vi "Pc Robo control.vi"() -> ()   [LabVIEW 2017]
uses:
  <vilib>/Utility/inputDevices.llb/joystickAcquire.vi
  <vilib>/Platform/NI_3dgraph.lvlib
panel:
  in  "error in (no error)":errorcluster
  in  "stop":bool
  out "error out":errorcluster
  out "Numeric":dbl
  out "Phi1":dbl
  out "K1":dbl
  out "Phi2":dbl
  out "K2":dbl
  out "L1":dbl(slide) scale=-0.09..0.09
  out "L2":dbl(slide) scale=-0.09..0.09
  out "L3":dbl(slide) scale=-0.09..0.09
  out "L4":dbl(slide) scale=-0.09..0.09
  out "L5":dbl(slide) scale=-0.09..0.09
  out "L6":dbl(slide) scale=-0.09..0.09
  in  "3D Curve":refnum<k7>(container)
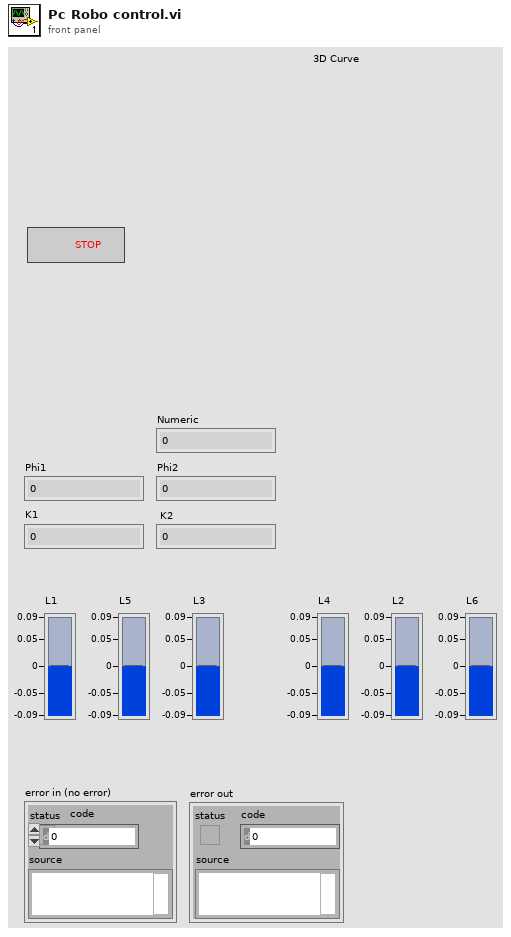
[diagram p1: front panel]
types:
  T1 = cluster{"X axis":i32, "Y axis":i32, "Z axis":i32, "X axis rotation":i32, "Y axis rotation":i32, "Z axis rotation":i32, "U axis":i32, "V axis":i32}
  T2 = cluster{"button 1":bool, "button 2":bool, "button 3":bool, "button 4":bool, "button 5":bool, "button 6":bool, "button 7":bool, "button 8":bool, "button 9":bool, "button 10":bool, "button 11":bool, "button 12":bool, "button 13":bool, "button 14":bool, "button 15":bool, "button 16":bool, "button 17":bool, "button 18":bool, "button 19":bool, "button 20":bool, "button 21":bool, "button 22":bool, "button 23":bool, "button 24":bool, "button 25":bool, "button 26":bool, "button 27":bool, "button 28":bool, "button 29":bool, "button 30":bool, "button 31":bool, "button 32":bool}
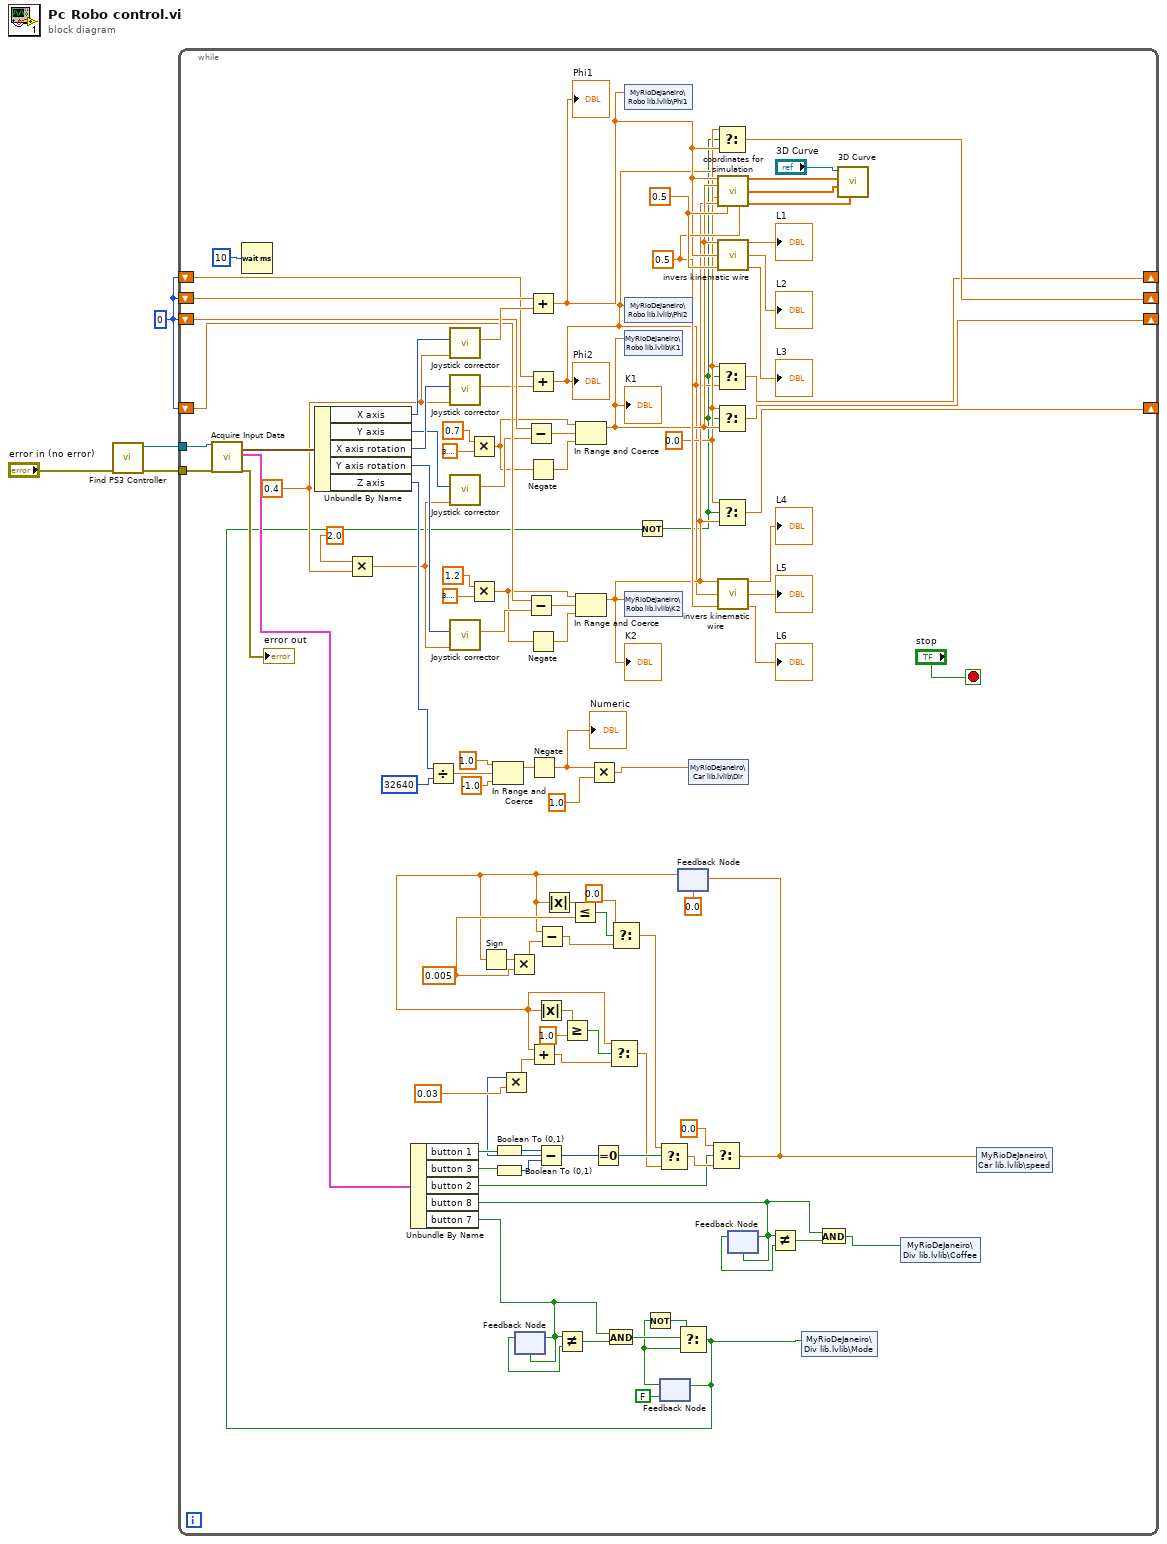
[diagram p0: block diagram]
diagram:
  w4 = 0
  n1 = call "Find PS3 Controller.vi"("error in (no error)"="error in (no error)") -> ("error out"=w2:errorcluster, "Controller Reference Out"=w3:refnum<k1>)  [unwired: 9 in]
  n2 = while {
    tunnel: w2 -> [w101]
    tunnel: w3 -> [w102]
    shift-right: [w60] -> _
    shift-left: w4 -> [w90]
    shift-right: [w57] -> _
    shift-left: w4 -> [w86]
    shift-right: [w59] -> _
    shift-left: w4 -> [w85]
    shift-right: [w55] -> _
    shift-left: w4 -> [w84]
    stop <- "stop" stop-if-true
    w65 = 0.4 ("rate")
    w33 = 0.005
    w67 = 0.5 ("S2")
    w71 = 0.5 ("S1")
    w54 = 0.0
    n3 = call-poly <vilib>:"Acquire Input Data.vi"("device ID"=w102, "error in (no error)"=w101) -> ("axis info"=w103:T1, "button info"=w48:T2, "error out"=→"error out":errorcluster)  [unwired: 15 out]
    n4 = Wait (ms)(milliseconds to wait=u32 10) -> ()  [unwired: 1 out]
    n5 = Unbundle By Name(w103) -> ("X axis"=w91:i32, "Y axis"=w92:i32, "X axis rotation"=w93:i32, "Y axis rotation"=w94:i32, "Z axis"=w99:i32)
    n6 = Multiply(x=2.0 ("c-rate"), y=w65) -> (x*y=w66:dbl)
    n7 = Unbundle By Name(w48) -> ("button 1"=w44:bool, "button 3"=w43:bool, "button 2"=w19:bool, "button 8"=w15:bool, "button 7"=w11:bool)
    n8 = Divide(x=w99, y=32640) -> (x/y=w96:dbl)
    n9 = call "Joystick corrector.vi"("rate"=w65, "Joystick"=w91) -> ("output"=w89:dbl)  [unwired: 9 in]
    n10 = call "Joystick corrector.vi"("rate"=w65, "Joystick"=w93) -> ("output"=w82:dbl)  [unwired: 9 in]
    n11 = call "Joystick corrector.vi"("rate"=w66, "Joystick"=w92) -> ("output"=w81:dbl)  [unwired: 9 in]
    n12 = call "Joystick corrector.vi"("rate"=w66, "Joystick"=w94) -> ("output"=w83:dbl)  [unwired: 9 in]
    n13 = Multiply(x=0.7 ("upper limit"), y=3.141592653589793) -> (x*y=w51:dbl)
    n14 = Multiply(x=1.2 ("upper limit"), y=3.141592653589793) -> (x*y=w62:dbl)
    n15 = In Range and Coerce(upper limit=1.0, x=w96, lower limit=-1.0) -> (coerced(x)=w95:dbl)  [unwired: 1 out]
    n16 = Boolean To (0,1)(Boolean=w44) -> (0, 1=w42:i16)
    n17 = Boolean To (0,1)(Boolean=w43) -> (0, 1=w41:i16)
    n18 = feedback #1(w11) -> (w13:bool)
    n19 = feedback-in #1(w11) -> ()
    n20 = Subtract(x=w86, y=w81) -> (x-y=w80:dbl)
    n21 = Subtract(x=w84, y=w83) -> (x-y=w79:dbl)
    n22 = Add(x=w90, y=w89) -> (x+y=w61:dbl)
    "Phi1" <- w61
    n23 = Add(x=w85, y=w82) -> (x+y=w49:dbl)
    "Phi2" <- w49
    n24 = Negate(x=w51) -> (-x=w50:dbl)
    n25 = Negate(x=w62) -> (-x=w63:dbl)
    n26 = Negate(x=w95) -> (-x=w47:dbl)
    "Numeric" <- w47
    n27 = Subtract(x=w42, y=w41) -> (x-y=w25:i16)
    n28 = Multiply(x=w25, y=0.03) -> (x*y=w30:dbl)
    n29 = Not Equal?(x=w11, y=w13) -> (x != y?=w12:bool)
    n30 = In Range and Coerce(upper limit=w51, x=w80, lower limit=w50) -> (coerced(x)=w58:dbl)  [unwired: 1 out]
    "K1" <- w58
    n31 = In Range and Coerce(upper limit=w62, x=w79, lower limit=w63) -> (coerced(x)=w56:dbl)  [unwired: 1 out]
    "K2" <- w56
    n32 = Multiply(x=w47, y=1.0) -> (x*y=w45:dbl)
    n33 = Equal To 0?(x=w25) -> (x = 0?=w40:bool)
    n34 = And(x=w11, y=w12) -> (x .and. y?=w10:bool)
    n35 = shared-variable "MyRioDeJaneiro\\Robo lib.lvlib\\Phi1"(w61) -> ()  [unwired: 1 in, 1 out]
    n36 = shared-variable "MyRioDeJaneiro\\Robo lib.lvlib\\Phi2"(w49) -> ()  [unwired: 1 in, 1 out]
    n37 = shared-variable "MyRioDeJaneiro\\Robo lib.lvlib\\K1"(w58) -> ()  [unwired: 1 in, 1 out]
    n38 = shared-variable "MyRioDeJaneiro\\Robo lib.lvlib\\K2"(w56) -> ()  [unwired: 1 in, 1 out]
    n39 = feedback #2(FALSE) -> (w8:bool)
    n40 = Not(x=w8) -> (.not. x?=w9:bool)
    n41 = feedback #3(0.0) -> (w22:dbl)
    n42 = Sign(1:w22) -> (0:w39:dbl)
    n43 = Multiply(x=w39, y=w33) -> (x*y=w38:dbl)
    n44 = Add(x=w22, y=w30) -> (x+y=w28:dbl)
    n45 = Absolute Value(x=w22) -> (abs(x)=w26:dbl)
    n46 = Subtract(x=w22, y=w38) -> (x-y=w34:dbl)
    n47 = Absolute Value(x=w22) -> (abs(x)=w32:dbl)
    n48 = Greater Or Equal?(x=w26, y=1.0) -> (x >= y?=w29:bool)
    n49 = Less Or Equal?(x=w32, y=w33) -> (x <= y?=w35:bool)
    n50 = Select(t=w22, s=w29, f=w28) -> (s? t:f=w23:dbl)
    n51 = Select(t=0.0, s=w35, f=w34) -> (s? t:f=w36:dbl)
    n52 = Select(t=w36, s=w40, f=w23) -> (s? t:f=w21:dbl)
    n53 = Select(t=w9, s=w10, f=w8) -> (s? t:f=w5:bool)
    n54 = Not(x=w5) -> (.not. x?=w6:bool)
    n55 = feedback-in #2(w5) -> ()
    n56 = shared-variable "MyRioDeJaneiro\\Car lib.lvlib\\Dir"(w45) -> ()  [unwired: 1 in, 1 out]
    n57 = Select(t=0.0, s=w19, f=w21) -> (s? t:f=w18:dbl)
    n58 = feedback-in #3(w18) -> ()
    n59 = Select(t=w54, s=w6, f=w61) -> (s? t:f=w60:dbl)
    n60 = Select(t=w54, s=w6, f=w49) -> (s? t:f=w59:dbl)
    n61 = Select(t=w54, s=w6, f=w58) -> (s? t:f=w57:dbl)
    n62 = Select(t=w54, s=w6, f=w56) -> (s? t:f=w55:dbl)
    n63 = call "coordinates for simulation.vi"("phi1"=w61, "k1"=w58, "phi2"=w49, "k2"=w56, "s1"=w71, "s2"=w67) -> ("X"=w78:dbl[], "Y"=w77:dbl[], "Z"=w76:dbl[])  [unwired: 7 in]
    n64 = call "invers kinematic wire.vi"("K"=w58, "phi"=w61, "s"=w71) -> ("L1"=→"L1":dbl, "L 2"=→"L2":dbl, "L 3"=→"L3":dbl)  [unwired: 10 in]
    n65 = call "invers kinematic wire.vi"("K"=w56, "phi"=w49, "s"=w67) -> ("L1"=→"L4":dbl, "L 2"=→"L5":dbl, "L 3"=→"L6":dbl)  [unwired: 10 in]
    n66 = feedback-in #4(w15) -> ()
    n67 = feedback #4(w15) -> (w17:bool)
    n68 = Not Equal?(x=w15, y=w17) -> (x != y?=w16:bool)
    n69 = shared-variable "MyRioDeJaneiro\\Div lib.lvlib\\Mode"(w5) -> ()  [unwired: 1 in, 1 out]
    n70 = And(x=w15, y=w16) -> (x .and. y?=w14:bool)
    n71 = call <vilib>:"3D Curve.vi"("z vector"=w76, "y vector"=w77, "x vector"=w78, "3D graph"="3D Curve") -> ()  [unwired: 6 in, 2 out]
    n72 = shared-variable "MyRioDeJaneiro\\Div lib.lvlib\\Coffee"(w14) -> ()  [unwired: 1 in, 1 out]
    n73 = shared-variable "MyRioDeJaneiro\\Car lib.lvlib\\speed"(w18) -> ()  [unwired: 1 in, 1 out]
  }
